vi "控件的属性和方法.vi"() -> ()   [LabVIEW 2022 SP3]
doc: "本VI是为《我和LabVIEW》一书编写的示例。\n关于本书的介绍请参考网页：\nhttp://ruanqizhen.spaces.live.com/blog/cns!5852D4F797C53FB6!4310.entry"
panel:
  in  "数值":dbl
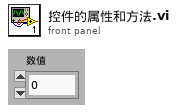
[diagram p1: front panel]
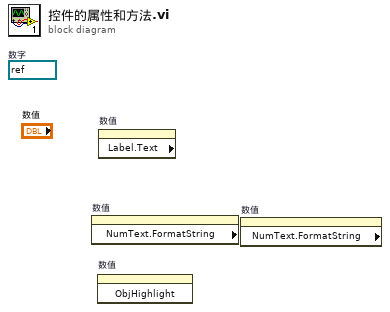
[diagram p0: block diagram]
diagram:
  (unwired) refnum<vi> refnum  # 数字
  n1 = property on="数值" class="DigNum (严格)" props=["NumText", "FormatString"]() -> ()  [unwired: 2 in, 3 out]
  n2 = invoke on="数值" class="DigNum (严格)" method="ObjHighlight"() -> ()  [unwired: 3 in, 3 out]
  n3 = property on="数值" class="DigNum (严格)" props=["Label", "Text"]() -> ()  [unwired: 2 in, 3 out]
  n4 = property on="数值" class="数字 (严格)" props=["NumText", "FormatString"]() -> ()  [unwired: 2 in, 3 out]
